vi "SingleMeasurement.vi"(8 "error in (no error)":errorcluster, 11 "VISA resource name":refnum<visa-resource-name>) -> (0 "error out":errorcluster, 2 "output / s":dbl, 3 "VISA resource name out":refnum<visa-resource-name>)   [LabVIEW 2018, in "GP22_TDC_Arduinoed.lvlib"]
doc: "Take a single TDC measurement.\n\nIf the GP22 is not set to automatically calibrate on every run, perform a TDC calibration before the measurement."
uses:
  GP22_TDC_Arduinoed.lvlib
  Private/ConvertTimes - Single.vi
panel:
  out "read buffer":string
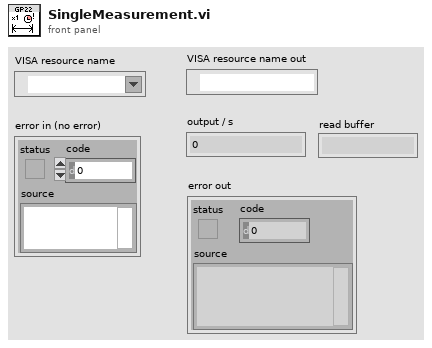
[diagram p1: front panel]
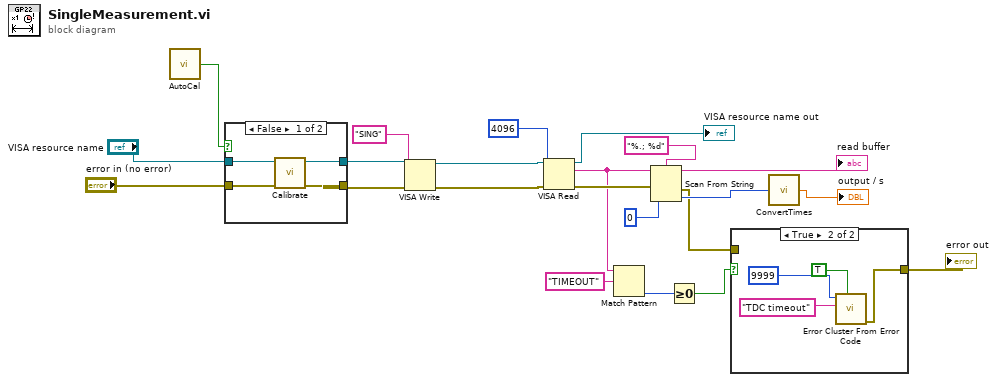
[diagram p0: block diagram]
diagram:
  n1 = call "AutoCal.vi"() -> ("Autocal mode?"=w1:bool)  [unwired: 2 in]
  n2 = case shown="False" w1 {
    tunnel: "VISA resource name" -> [w25 w27]
    tunnel: "error in (no error)" -> [w24 w26]
    tunnel: [w23 w26] -> w13
    tunnel: [w22 w27] -> w10
    frame False {
      n3 = call "Calibrate.vi"("error in (no error)"=w24, "VISA resource name"=w25) -> ("error out"=w23:errorcluster, "VISA resource name out"=w22:refnum<visa-resource-name>)  [unwired: 5 in, 2 out]
    }
    frame True {
    }
  }
  n4 = VISA Write(VISA resource name=w10, write buffer="SING" ("command"), error in (no error)=w13) -> (VISA resource name out=w9:refnum<visa-resource-name>, error out=w8:errorcluster)  [unwired: 1 out]
  n5 = VISA Read(VISA resource name=w9, byte count=u32 4096, error in (no error)=w8) -> (VISA resource name out=→"VISA resource name out":refnum<visa-resource-name>, read buffer=w3:string, error out=w18:errorcluster)  [unwired: 1 out]
  "read buffer" <- w3
  n6 = Match Pattern(string=w3, regular expression="TIMEOUT") -> (offset past match=w5:i32)  [unwired: 1 in, 3 out]
  n7 = Scan From String(format string="%.; %d", input string=w3, error in=w18, default 1=u32 0 ("default value 1")) -> (error out=w6:errorcluster, output 1=w16:u32)  [unwired: 1 in, 2 out]
  n8 = Greater Or Equal To 0?(x=w5) -> (x >= 0?=w4:bool)
  n9 = case shown="True" w4 {
    tunnel: [w28 w29] -> w7
    tunnel: w6 -> [w28 _]
    frame False {
    }
    frame True {
      n10 = call <vilib>:"Error Cluster From Error Code.vi"("show call chain? (False)"=TRUE, "error message (\"\")"="TDC timeout" ("source"), "error code (0)"=9999 ("code")) -> ("error out"=w29:errorcluster)  [unwired: 6 in]
    }
  }
  "error out" <- w7
  n11 = call-poly "ConvertTimes.vi"("GP22 Output"=w16) -> ("Time/s"=→"output / s":dbl)
